vi "hidSPD Close Session.vi"(8 "error in (no error)":errorcluster, 11 "spdDevHandle":T1) -> (0 "error out":errorcluster)   [LabVIEW 2018, in "hidSPDLibForLabView.lvlib"]
uses:
  hidSPDLibForLabView.lvlib
  hidSPD Controls/hidSPD Device Session.ctl
  <vilib>/Utility/error.llb/Error Cluster From Error Code.vi
  <vilib>/ErrorRing/Error Ring.xnode
  hidSPD DLL files/libSPD.dll
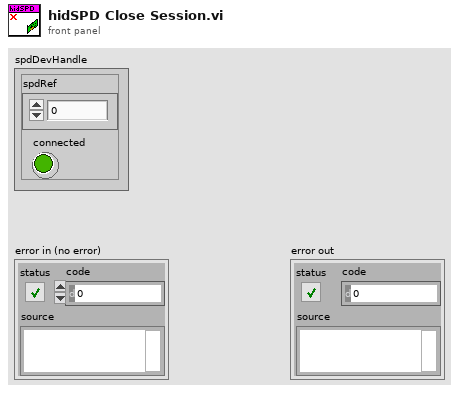
[diagram p1: front panel]
types:
  T1 = typedef "hidSPDLibForLabView.lvlib/hidSPD Device Session.ctl" = cluster{"spdRef":u64, "connected":bool}
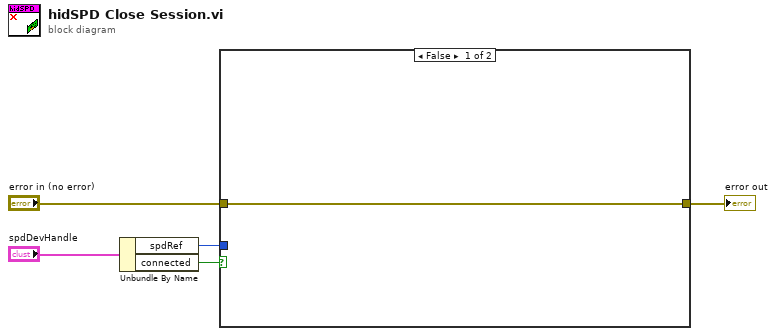
[diagram p0: block diagram]
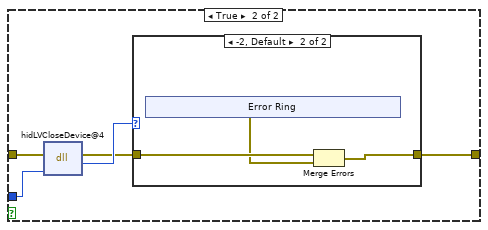
[diagram p2: hidden frame]
diagram:
  n1 = Unbundle By Name("spdDevHandle") -> ("spdRef"=w2:u64, "connected"=w1:bool)
  n2 = case shown="False" w1 {
    tunnel: "error in (no error)" -> [w6 w11]
    tunnel: [w6 w8] -> w4
    tunnel: w2 -> [_ w7]
    frame False {
    }
    frame True {
      n3 = dll-call lib="D:/NextCloud/SPD stand/Automative SPD Measurements/Automative SPD Stand/Instruments/SPD HID Interface/hidSPDLibForLabView/hidSPD DLL files/libSPD.dll" fn="hidLVCloseDevice@4"(error in=w11, "spdDevHandle"=w7) -> (error out=w9:errorcluster, "errorCode"=w10:i32)  [unwired: 3 in, 1 out]
      n4 = case shown="-2, Default" w10 {
        tunnel: w9 -> [w12 w15]
        tunnel: [w12 w13] -> w8
        frame 0 {
        }
        frame -2, Default {
          n5 = xnode "Error Ring"() -> ("error out"=w14:errorcluster)
          n6 = Merge Errors(w15, w14) -> (w13:errorcluster)
        }
      }
    }
  }
  "error out" <- w4
